vi "VI Control - Set Front Panel Colour.vi"(0 "VI Path":path, 7 "Front Panel Colour":u32(colorbox)) -> (15 "error out":errorcluster)   [LabVIEW 2011]
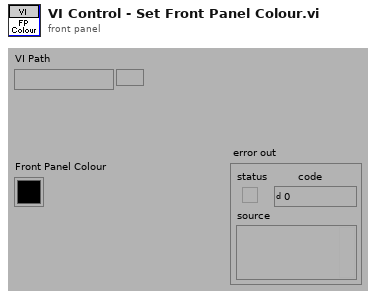
[diagram p1: front panel]
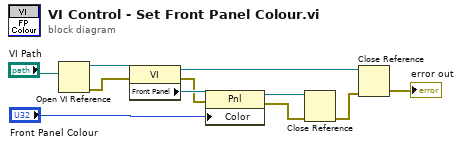
[diagram p0: block diagram]
diagram:
  n1 = Open VI Reference(vi path="VI Path") -> (vi reference=w11:refnum<vi>, error out=w8:errorcluster)  [unwired: 5 in]
  n2 = property class="VI"(reference=w11, error in=w8) -> (reference out=w3:refnum<vi>, error out=w7:errorcluster, "Front Panel"=w10:refnum<vi>)
  n3 = property class="Pnl"(reference=w10, error in=w7, "Color"="Front Panel Colour") -> (reference out=w5:refnum<vi>, error out=w6:errorcluster)
  n4 = Close Reference(reference=w5, error in (no error)=w6) -> (error out=w4:errorcluster)
  n5 = Close Reference(reference=w3, error in (no error)=w4) -> (error out=→"error out":errorcluster)
